vi "Filename.vi"(8 "error in (no error)":errorcluster, 9 "P Graph and Intensities and RF":cluster{"Array":dbl[], "Array":dbl[]}[](array[cluster]), 10 "Q Graph":cluster{"Array":dbl[], "Array 2":dbl[]}, 11 "Byte Stream File in":refnum<file>) -> (0 "error out":errorcluster, 3 "Byte Stream File out":refnum<file>)   [LabVIEW 2018]
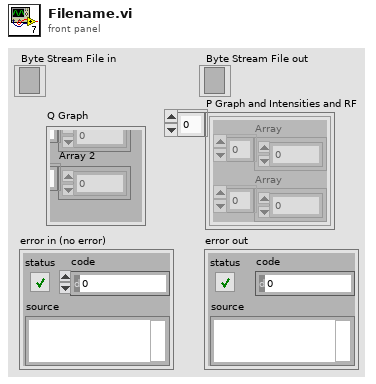
[diagram p1: front panel]
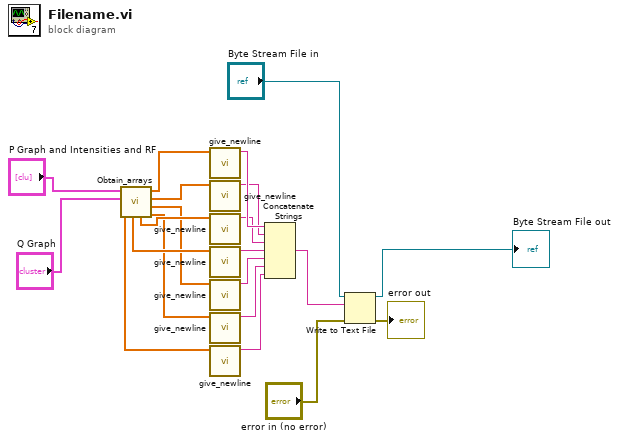
[diagram p0: block diagram]
diagram:
  n1 = call "Obtain_arrays.vi"("Q Graph"="Q Graph", "P Graph and Intensities and RF"="P Graph and Intensities and RF") -> ("RF Range 2"=w2:dbl[], "RF Range 1"=w3:dbl[], "Q"=w6:dbl[], "P"=w7:dbl[], "I+"=w5:dbl[], "I-"=w4:dbl[], "AFP Range"=w1:dbl[])  [unwired: 3 in]
  n2 = call "give_newline.vi"("Array for writing"=w7) -> ("To file with newline"=w14:string)  [unwired: 10 in]
  n3 = call "give_newline.vi"("Array for writing"=w6) -> ("To file with newline"=w13:string)  [unwired: 10 in]
  n4 = call "give_newline.vi"("Array for writing"=w5) -> ("To file with newline"=w12:string)  [unwired: 10 in]
  n5 = call "give_newline.vi"("Array for writing"=w4) -> ("To file with newline"=w11:string)  [unwired: 10 in]
  n6 = call "give_newline.vi"("Array for writing"=w3) -> ("To file with newline"=w10:string)  [unwired: 10 in]
  n7 = call "give_newline.vi"("Array for writing"=w2) -> ("To file with newline"=w9:string)  [unwired: 10 in]
  n8 = call "give_newline.vi"("Array for writing"=w1) -> ("To file with newline"=w8:string)  [unwired: 10 in]
  n9 = Concatenate Strings(w14, w13, w12, w11, w10, w9, w8) -> (w15:string)
  n10 = Write to Text File(file (use dialog)="Byte Stream File in", text=w15, error in="error in (no error)") -> (refnum out=→"Byte Stream File out":refnum<file>, error out=→"error out":errorcluster)  [unwired: 1 in, 1 out]
